vi "Configure Control Parameters.vi"(0 "VISA resource name":refnum<visa-resource-name>, 1 "Manual Output (0.000 %)":dbl min=0.0 max=100.0 step=0.001 format="%.3f", 2 "Heater Range (0: Off)":u16(ring) items=["Off", "Low (0.5W)", "Med (5W)", "High (50W)"], 5 "Loop (0: 1)":u16(ring) items=["1", "2"], 7 "Gain (P) (0.0)":dbl min=0.0 max=1000.0 step=0.1 format="%.1f", 9 "Reset (I) (0.0)":dbl min=0.0 max=1000.0 step=0.1 format="%.1f", 11 "error in (no error)":errorcluster, 12 "Rate (D) (0)":dbl min=0.0 max=200.0 step=1.0) -> (4 "VISA resource name out":refnum<visa-resource-name>, 15 "error out":errorcluster)   [LabVIEW 2013, in "Lake Shore Cryotronics 331.lvlib"]
doc: "This VI Configures the 331 Control Parameters for the selected loop, functions configured are PID, Heater Range, and Manual Output."
uses:
  Lake Shore Cryotronics 331.lvlib
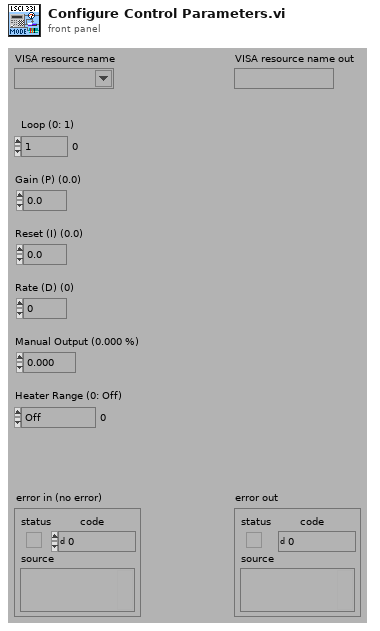
[diagram p1: front panel]
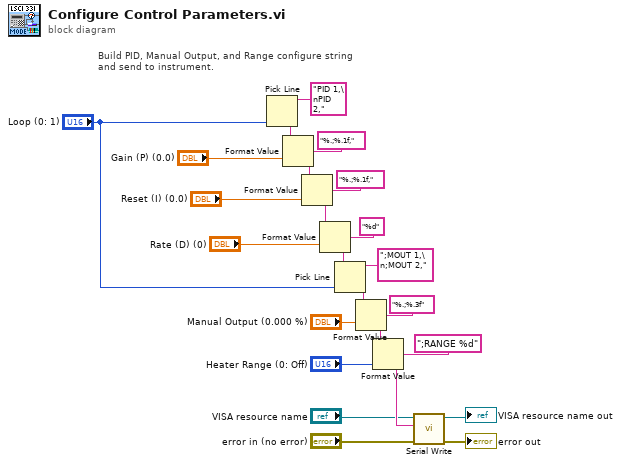
[diagram p0: block diagram]
diagram:
  # "Build PID, Manual Output, and Range configure string\nand send to instrument."
  n1 = Pick Line(multi-line string="PID 1,\nPID 2,", line index="Loop (0: 1)") -> (output string=w19:string)  [unwired: 1 in]
  n2 = Format Value(string ("")=w19, format string="%.;%.1f,", value (0)="Gain (P) (0.0)") -> (output string=w18:string)
  n3 = Format Value(string ("")=w18, format string="%.;%.1f,", value (0)="Reset (I) (0.0)") -> (output string=w17:string)
  n4 = Format Value(string ("")=w17, format string="%d", value (0)="Rate (D) (0)") -> (output string=w12:string)
  n5 = Pick Line(string ("")=w12, multi-line string=";MOUT 1,\n;MOUT 2,", line index="Loop (0: 1)") -> (output string=w8:string)
  n6 = Format Value(string ("")=w8, format string="%.;%.3f", value (0)="Manual Output (0.000 %)") -> (output string=w6:string)
  n7 = Format Value(string ("")=w6, format string=";RANGE %d", value (0)="Heater Range (0: Off)") -> (output string=w5:string)
  n8 = call "Serial Write.vi"("error in (no error)"="error in (no error)", "Write Buffer (\"\")"=w5, "VISA resource name"="VISA resource name") -> ("error out"=→"error out":errorcluster, "VISA resource name out"=→"VISA resource name out":refnum<visa-resource-name>)  [unwired: 6 in, 1 out]
